vi "Analyze SPR data -- subVI.vi"(8 "error in (no error)":errorcluster, 9 "q Starting":dbl=40.0, 10 "Data":cluster{"Angle":dbl, "Data":dbl}[](array[cluster]), 11 "q Final":dbl=70.0) -> (0 "error out":errorcluster, 1 "q Middle":dbl, 2 "Minimun Intensity":dbl, 3 "qR":dbl, 4 "Curve width":dbl format="%#.3g", 5 "No. de datos":i32, 6 "Maximum Intensity":dbl, 7 "SPR Curve":cluster{"EJE X":dbl[], dbl[]}(graph))   [LabVIEW 2020]
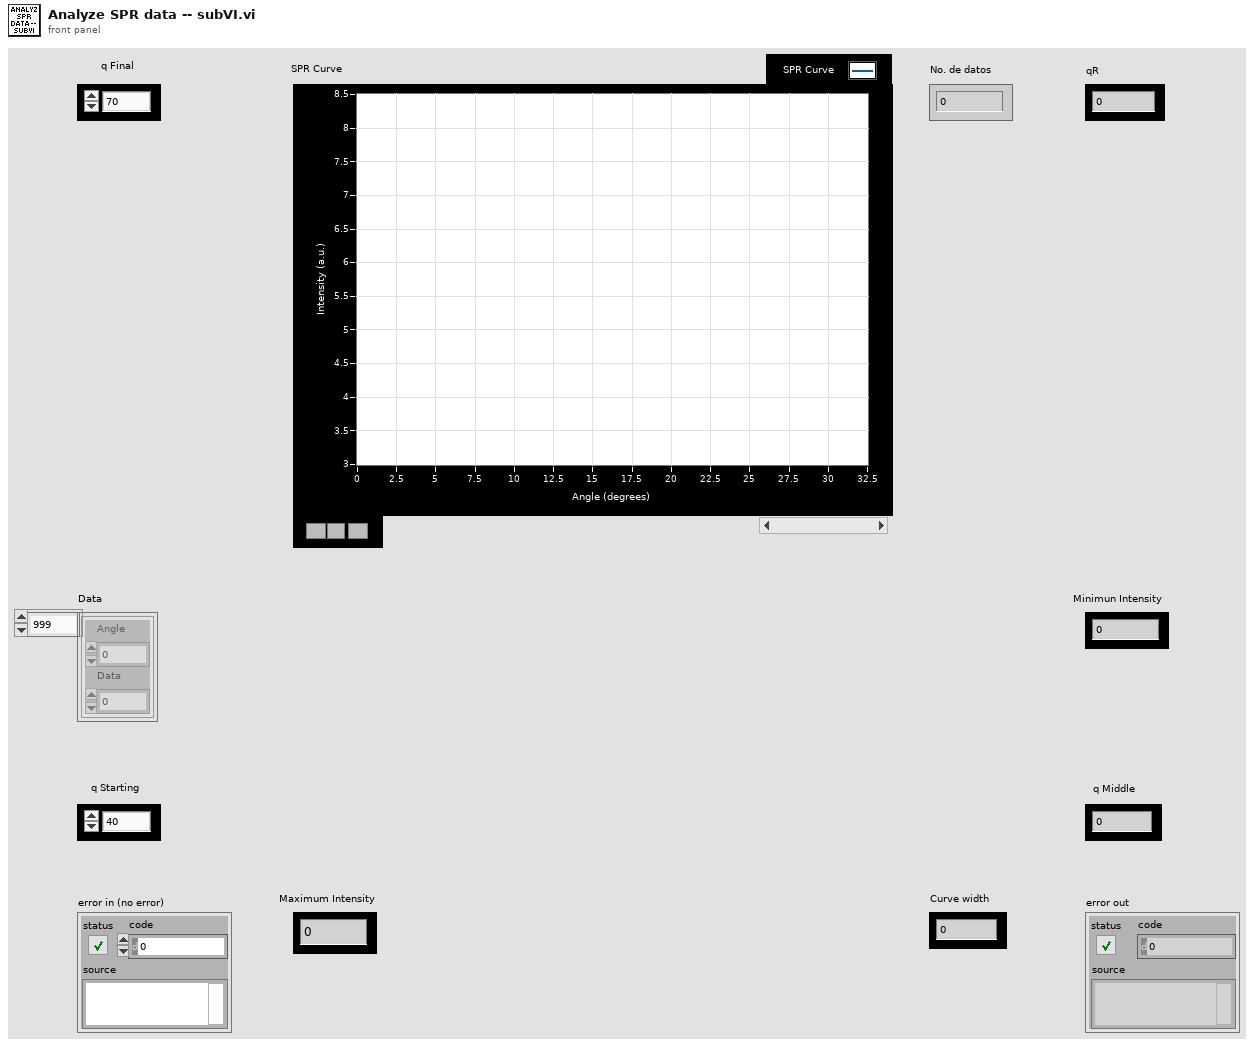
[diagram p1: front panel]
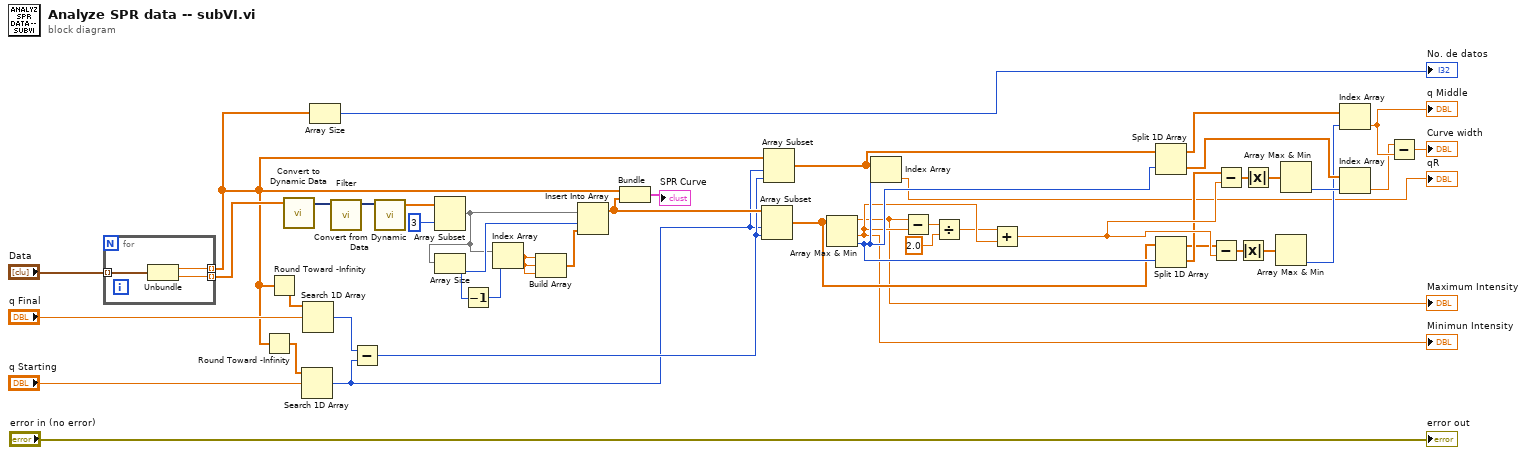
[diagram p0: block diagram]
diagram:
  n1 = for {
    tunnel: "Data" -> [w49] mode=indexing
    tunnel: [w48] -> w3 mode=indexing
    tunnel: [w47] -> w4 mode=indexing
    n2 = Unbundle(w49) -> ("Angle"=w48:dbl, "Data"=w47:dbl)
  }
  n3 = Round Toward -Infinity(1:w3) -> (0:w46:dbl[])
  n4 = Round Toward -Infinity(1:w3) -> (0:w45:dbl[])
  n5 = call "Convert to Dynamic Data"("Array"=w4) -> ("Dynamic Data Type"=w7:dynamicdata)  [unwired: 3 in]
  n6 = Search 1D Array(1D array=w46, element="q Starting") -> (index of element=w16:i32)  [unwired: 1 in]
  n7 = Search 1D Array(1D array=w45, element="q Final") -> (index of element=w6:i32)  [unwired: 1 in]
  n8 = Array Size(array=w3) -> (size(s)=→"No. de datos":i32)
  n9 = call "Filter"("Signal"=w7) -> ("Filtered Signal"=w8:dynamicdata)  [unwired: 9 in, 1 out]
  n10 = Subtract(x=w6, y=w16) -> (x-y=w17:i32)
  n11 = call "Convert from Dynamic Data"("Dynamic Data Type"=w8) -> ("Array"=w15:dbl[])  [unwired: 3 in]
  n12 = Array Subset(array=w15, index=3 ("length")) -> (w10:dbl[])  [unwired: 1 in]
  n13 = Array Size(array=w10) -> (size(s)=w13:i32)
  n14 = Decrement(x=w13) -> (x-1=w11:i32)
  n15 = Index Array(array=w10, index=w11) -> (element=w12:dbl)
  n16 = Build Array(w12, w12, w12) -> (w14:dbl[])
  n17 = Insert Into Array(array=w10, index=w13, new element=w14) -> (w19:dbl[])
  n18 = Bundle(w3, w19) -> (→"SPR Curve":cluster{dbl[], dbl[]})  [unwired: 1 in]
  n19 = Array Subset(array=w19, index=w16, length=w17) -> (w26:dbl[])
  n20 = Array Subset(array=w3, index=w16, length=w17) -> (w30:dbl[])
  n21 = Array Max & Min(array=w26) -> (max value=w21:dbl, min value=w25:dbl, min index (indices)=w34:i32)  [unwired: 1 out]
  "Minimun Intensity" <- w25
  "Maximum Intensity" <- w21
  n22 = Index Array(array=w30, index=w34) -> (element=→"qR":dbl)
  n23 = Subtract(x=w21, y=w25) -> (x-y=w22:dbl)
  n24 = Divide(x=w22, y=2.0) -> (x/y=w24:dbl)
  n25 = Add(x=w24, y=w25) -> (x+y=w38:dbl)
  n26 = Split 1D Array(array=w30, index=w34) -> (first subarray=w31:dbl[], second subarray=w33:dbl[])
  n27 = Split 1D Array(array=w26, index=w34) -> (first subarray=w27:dbl[], second subarray=w37:dbl[])
  n28 = Subtract(x=w27, y=w38) -> (x-y=w28:dbl[])
  n29 = Subtract(x=w37, y=w38) -> (x-y=w36:dbl[])
  n30 = Absolute Value(x=w28) -> (abs(x)=w29:dbl[])
  n31 = Absolute Value(x=w36) -> (abs(x)=w35:dbl[])
  n32 = Array Max & Min(array=w29) -> (min index (indices)=w32:i32)  [unwired: 3 out]
  n33 = Array Max & Min(array=w35) -> (min index (indices)=w39:i32)  [unwired: 3 out]
  n34 = Index Array(array=w31, index=w32) -> (element=w41:dbl)
  "q Middle" <- w41
  n35 = Index Array(array=w33, index=w39) -> (element=w40:dbl)
  n36 = Subtract(x=w40, y=w41) -> (x-y=→"Curve width":dbl)
  "error out" <- "error in (no error)"
